vi "initialize.vi"() -> ()   [LabVIEW 2013]
uses:
  Global 1.vi
panel:
  in  "Exit":bool
  in  "Run":bool
  in  "Do You Want To Clean The LivingRoom?":bool
  in  "Loading...":u8(slide) scale=0.0..5.0
  out "Total Time:":i32
  in  "Return To Home Position":bool
  in  "Y":dbl min=-200.0 max=200.0 step=1.0
  in  "X":dbl min=-200.0 max=200.0 step=1.0
  in  "Rooms":i32(slide) scale=1.0..8.0
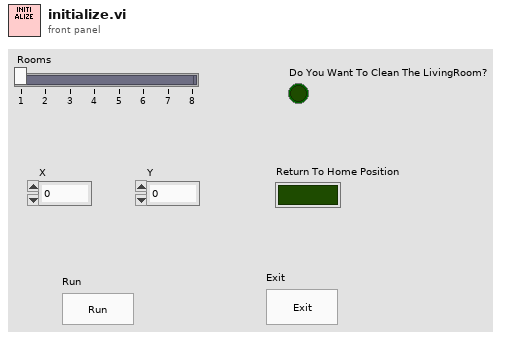
[diagram p1: front panel]
types:
  T1 = enum8{"Enabled", "Disabled", "Disabled and Grayed Out"}
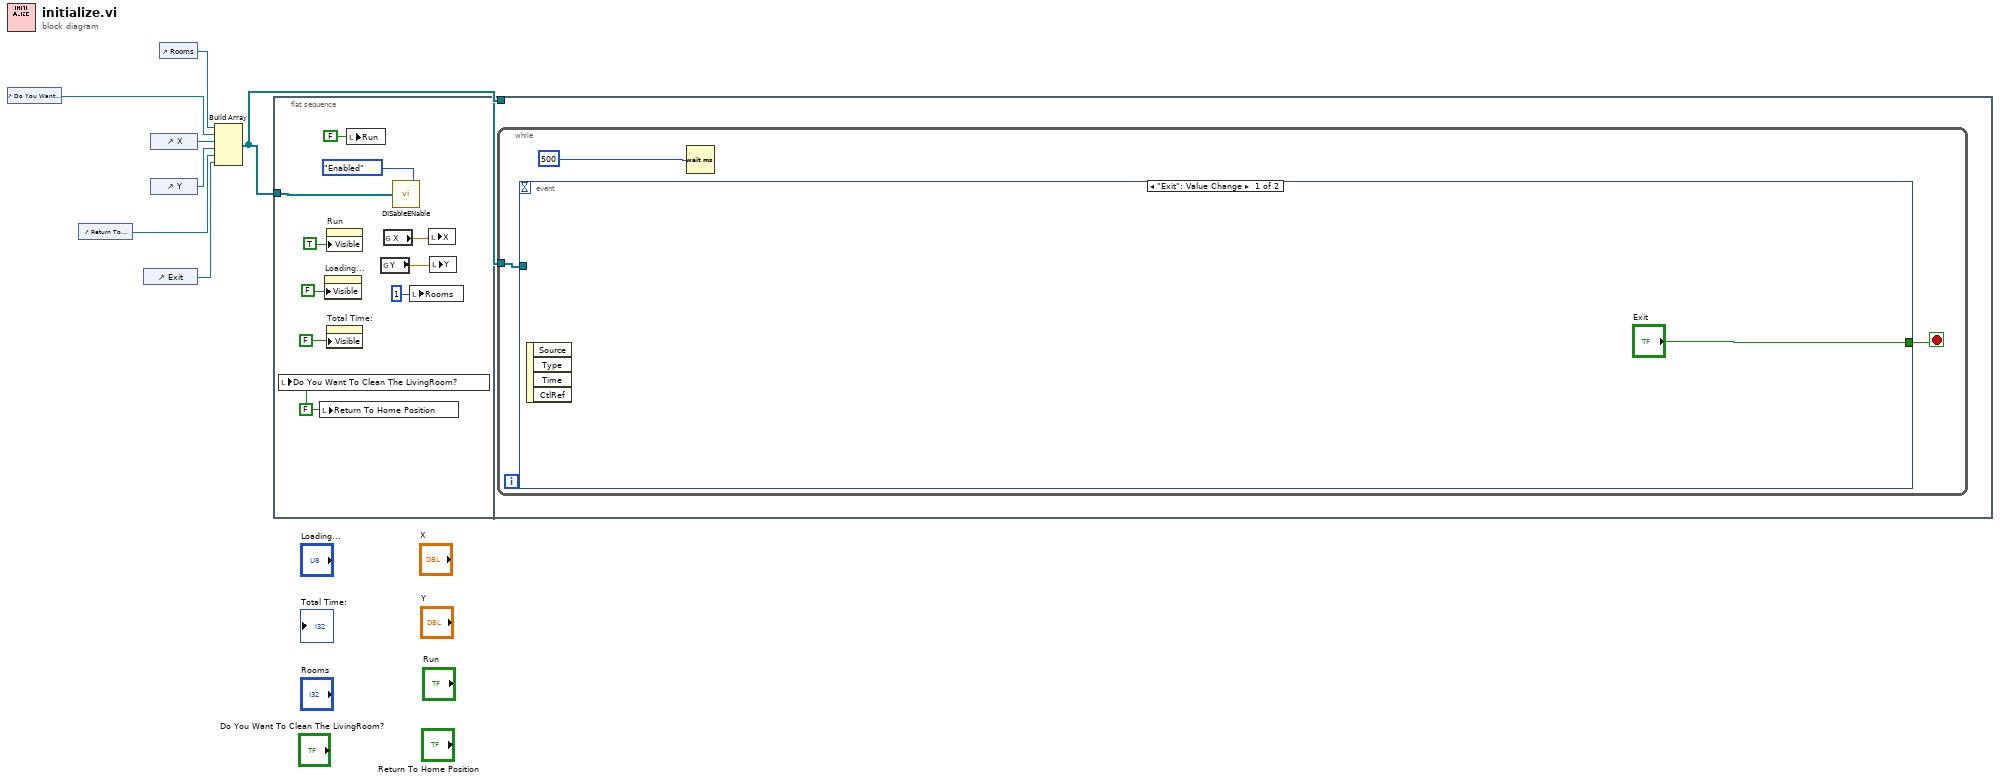
[diagram p0: block diagram]
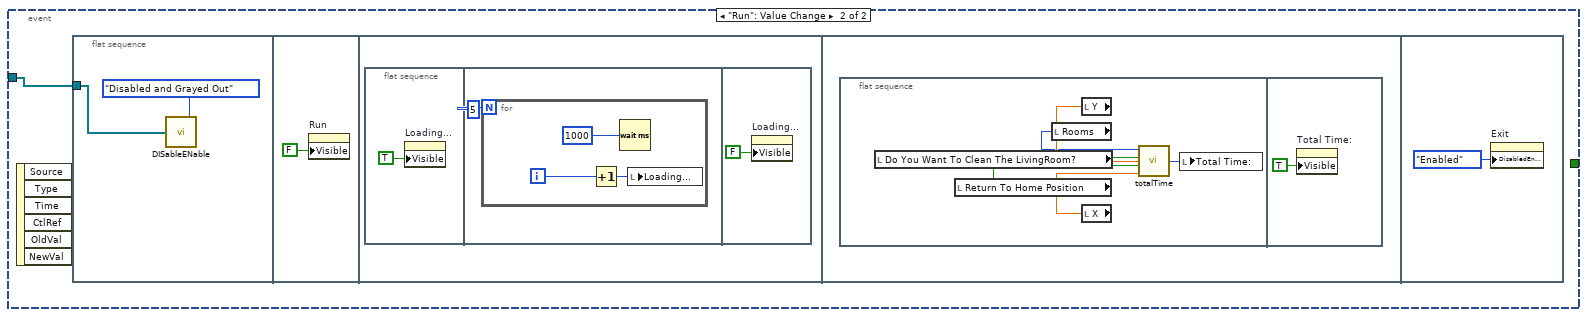
[diagram p2: hidden frame]
diagram:
  n1 = control-ref of="Do You Want To Clean The LivingRoom?"() -> (w3:refnum<vi>)
  n2 = control-ref of="Return To Home Position"() -> (w6:refnum<vi>)
  n3 = control-ref of="Exit"() -> (w7:refnum<vi>)
  n4 = control-ref of="X"() -> (w4:refnum<vi>)
  n5 = control-ref of="Y"() -> (w5:refnum<vi>)
  n6 = control-ref of="Rooms"() -> (w2:refnum<vi>)
  n7 = Build Array(w2, w3, w4, w5, w6, w7) -> (w1:refnum<vi>[])
  n8 = flat-sequence {
    tunnel: w1 -> [w13]
    tunnel: w1 -> [w18]
    frame #0 {
      w10 = FALSE ("Return To Home Position")
      n9 = local write "Do You Want To Clean The LivingRoom?"(w10) -> ()
      n10 = local write "Return To Home Position"(w10) -> ()
      n11 = property on="Loading..." class="Slide (strict)"("Visible"=FALSE) -> ()  [unwired: 2 in, 2 out]
      n12 = property on="Run" class="Bool (strict)"("Visible"=TRUE) -> ()  [unwired: 2 in, 2 out]
      n13 = property on="Total Time:" class="DigNum (strict)"("Visible"=FALSE) -> ()  [unwired: 2 in, 2 out]
      n14 = local write "Run"(FALSE ("Run")) -> ()
      n15 = global read "Global 1.vi" "Y"() -> (w9:dbl)
      n16 = global read "Global 1.vi" "X"() -> (w8:dbl)
      n17 = call "DISableENable.vi"("Disabled"=T1."Enabled", "Array"=w13) -> ()
      n18 = local write "Rooms"(1 ("Rooms")) -> ()
      n19 = local write "X"(w8) -> ()
      n20 = local write "Y"(w9) -> ()
    }
    frame #1 {
      n21 = while {
        tunnel: w18 -> [w20]
        stop <- w19 stop-if-true
        n22 = event shown="[0] \"Exit\": Value Change" {
          selector: _ -> [_ _]
          dyn-events: _ -> [_ _]
          timeout: _ -> [_ _]
          tunnel: w20 -> [_ w23]
          tunnel: ["Exit" _] -> w19
          event "Exit": Value Change {
            n23 = event-data() -> ()  [unwired: 1 in, 4 out]
          }
          event "Run": Value Change {
            n24 = event-data() -> ()  [unwired: 1 in, 6 out]
            n25 = flat-sequence {
              tunnel: w23 -> [w24]
              frame #0 {
                n26 = call "DISableENable.vi"("Disabled"=T1."Disabled and Grayed Out", "Array"=w24) -> ()
              }
              frame #1 {
                n27 = property on="Run" class="Bool (strict)"("Visible"=FALSE) -> ()  [unwired: 2 in, 2 out]
              }
              frame #2 {
                n28 = flat-sequence {
                  frame #0 {
                    n29 = property on="Loading..." class="Slide (strict)"("Visible"=TRUE) -> ()  [unwired: 2 in, 2 out]
                  }
                  frame #1 {
                    n30 = for {
                      N: 5 -> [_]
                      i -> [w30]
                      n31 = Increment(x=w30) -> (x+1=w29:i32)
                      n32 = Wait (ms)(milliseconds to wait=u32 1000 ("millisecond timer value")) -> ()  [unwired: 1 out]
                      n33 = local write "Loading..."(w29) -> ()
                    }
                  }
                  frame #2 {
                    n34 = property on="Loading..." class="Slide (strict)"("Visible"=FALSE) -> ()  [unwired: 2 in, 2 out]
                  }
                }
              }
              frame #3 {
                n35 = flat-sequence {
                  frame #0 {
                    n36 = local read "Do You Want To Clean The LivingRoom?"() -> (w36:bool)
                    n37 = local read "Return To Home Position"() -> (w35:bool)
                    n38 = local read "Rooms"() -> (w37:i32)
                    n39 = local read "Y"() -> (w38:dbl)
                    n40 = local read "X"() -> (w34:dbl)
                    n41 = call "totalTime.vi"("Rooms"=w37, "Do You Want To Clean The LivingRoom?"=w36, "Return To Home Position"=w35, "X"=w34, "Y"=w38) -> ("Total Time:"=w33:i32)
                    n42 = local write "Total Time:"(w33) -> ()
                  }
                  frame #1 {
                    n43 = property on="Total Time:" class="DigNum (strict)"("Visible"=TRUE) -> ()  [unwired: 2 in, 2 out]
                  }
                }
              }
              frame #4 {
                n44 = property on="Exit" class="Bool"("DisabledEnum"=T1."Enabled" ("Disabled")) -> ()  [unwired: 2 in, 2 out]
              }
            }
          }
        }
        n45 = Wait (ms)(milliseconds to wait=u32 500 ("millisecond timer value")) -> ()  [unwired: 1 out]
      }
    }
  }
